vi "Format Measurement Name and SG Pins.vi"(11 "Test Script In":string) -> (0 "Standard":string, 1 "SA Pin":string, 2 "SG Pin":string, 3 "Measurement Name Out":string, 4 "Band":string)   [LabVIEW 2016, in "QPA TCF Parser.lvlib" / "QPA TCF Parser.lvclass"]
uses:
  QPA TCF Parser.lvclass
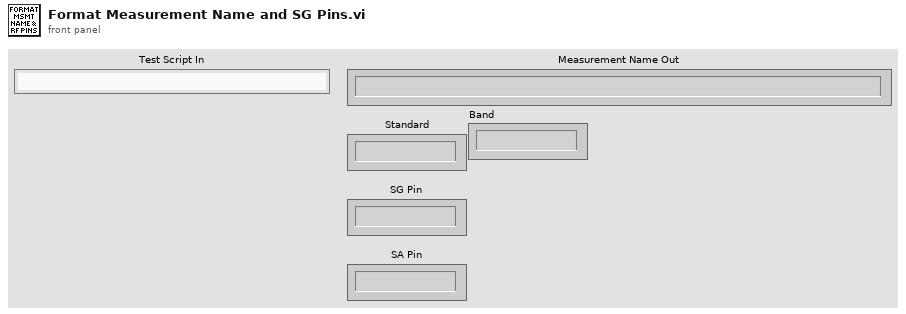
[diagram p1: front panel]
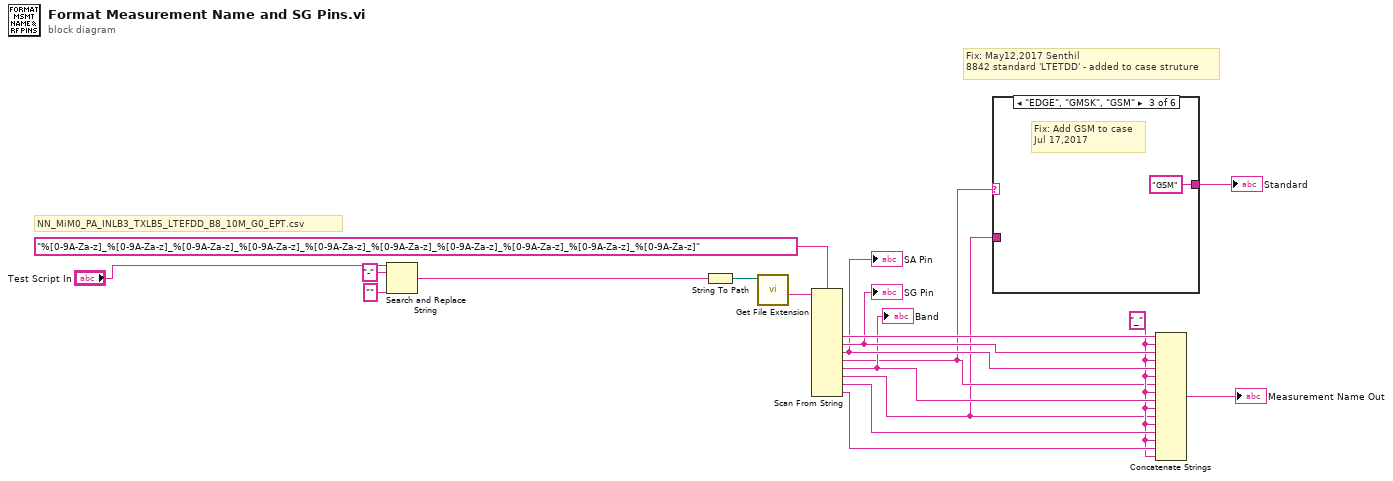
[diagram p0: block diagram]
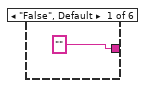
[diagram p2: hidden frame]
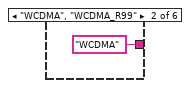
[diagram p3: hidden frame]
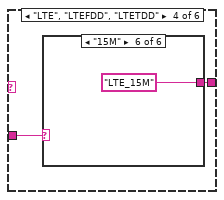
[diagram p4: hidden frame]
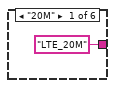
[diagram p5: hidden frame]
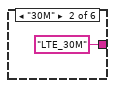
[diagram p6: hidden frame]
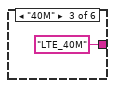
[diagram p7: hidden frame]
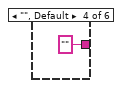
[diagram p8: hidden frame]
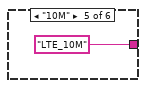
[diagram p9: hidden frame]
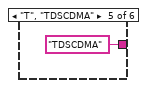
[diagram p10: hidden frame]
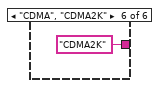
[diagram p11: hidden frame]
diagram:
  w9 = "_"
  # "Fix: May12,2017 Senthil\n8842 standard 'LTETDD' - added to case struture"
  # "NN_MiM0_PA_INLB3_TXLB5_LTEFDD_B8_10M_G0_EPT.csv"
  n1 = Search and Replace String(input string="Test Script In", search string="-", replace string="" ("replace string (\"\")")) -> (result string=w4:string)  [unwired: 5 in, 3 out]
  n2 = String To Path(string=w4) -> (path=w17:path)
  n3 = call <vilib>:"Get File Extension.vi"("file"=w17) -> ("filename without extension"=w18:string)  [unwired: 6 in, 4 out]
  n4 = Scan From String(format string="%[0-9A-Za-z]_%[0-9A-Za-z]_%[0-9A-Za-z]_%[0-9A-Za-z]_%[0-9A-Za-z]_%[0-9A-Za-z]_%[0-9A-Za-z]_%[0-9A-Za-z]_%[0-9A-Za-z]_%[0-9A-Za-z]", input string=w18) -> (output 3=w15:string, output 4=w14:string, output 5=w13:string, output 6=w7:string, output 7=w12:string, output 8=w5:string, output 9=w11:string, output 10=w10:string)  [unwired: 14 in, 3 out]
  "SG Pin" <- w14
  "SA Pin" <- w13
  "Band" <- w12
  n5 = case shown="\"EDGE\", \"GMSK\", \"GSM\"" w7 {
    tunnel: ["" "WCDMA" "GSM" w23 "TDSCDMA" "CDMA2K"] -> w6
    tunnel: w5 -> [_ _ _ w22 _ _]
    frame "False", Default {
    }
    frame "WCDMA", "WCDMA_R99" {
    }
    frame "EDGE", "GMSK", "GSM" {
      # "Fix: Add GSM to case\nJul 17,2017"
    }
    frame "LTE", "LTEFDD", "LTETDD" {
      n6 = case shown="\"15M\"" w22 {
        tunnel: ["LTE_20M" "LTE_30M" "LTE_40M" "" "LTE_10M" "LTE_15M"] -> w23
        frame "20M" {
        }
        frame "30M" {
        }
        frame "40M" {
        }
        frame "", Default {
        }
        frame "10M" {
        }
        frame "15M" {
        }
      }
    }
    frame "T", "TDSCDMA" {
    }
    frame "CDMA", "CDMA2K" {
    }
  }
  "Standard" <- w6
  n7 = Concatenate Strings(w15, w9, w14, w9, w13, w9, w7, w9, w12, w9, w5, w9, w11, w9, w10, w9) -> (→"Measurement Name Out":string)
